vi "Relay - Chan 1.vi"() -> ()   [LabVIEW 2022 SP3]
panel:
  out "standard output":string
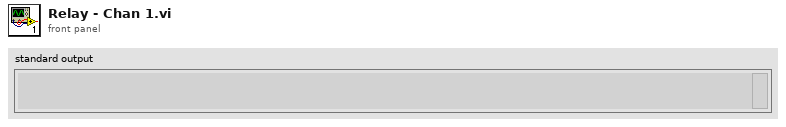
[diagram p1: front panel]
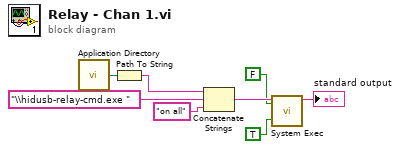
[diagram p0: block diagram]
diagram:
  n1 = call <vilib>:"Application Directory.vi"() -> ("Application Directory"=w3:path)
  n2 = Path To String(path=w3) -> (string=w2:string)
  n3 = Concatenate Strings(w2, "\\hidusb-relay-cmd.exe " ("command line"), "on all") -> (w7:string)
  n4 = call <vilib>:"System Exec.vi"("run minimized? (F)"=TRUE, "wait until completion? (T)"=FALSE, "command line"=w7) -> ("standard output"=→"standard output":string)  [unwired: 5 in, 3 out]
